vi "Cell colour.vi"() -> ()   [LabVIEW 2011]
uses:
  <vilib>/Utility/miscctls.llb/LVRowAndColumnTypeDef.ctl
panel:
  in  "Sub-Cycle Pattern":string[][](table) caption="Subcycle pattern"
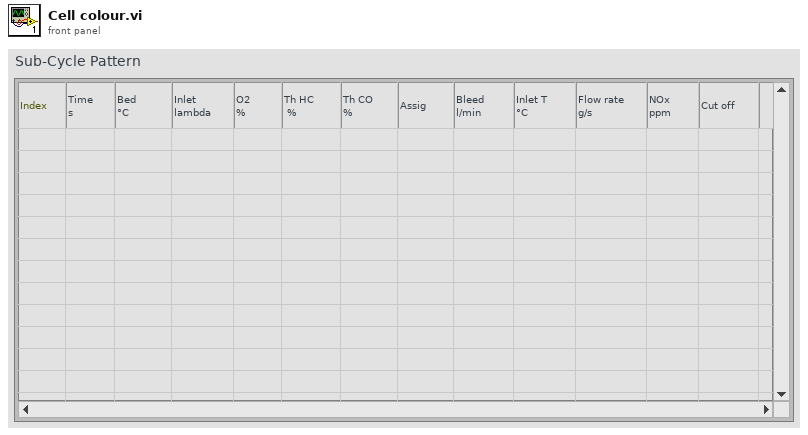
[diagram p1: front panel]
types:
  T1 = typedef "LVRowAndColumnTypeDef.ctl" = cluster{"Row":i32, "Column":i32}
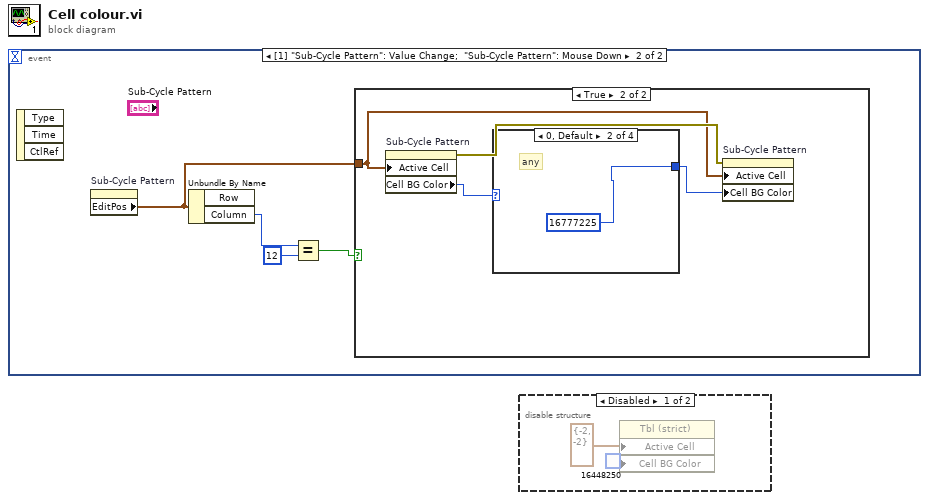
[diagram p0: block diagram]
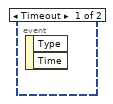
[diagram p3: hidden frame]
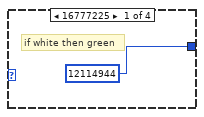
[diagram p5: hidden frame]
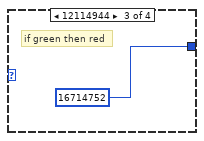
[diagram p6: hidden frame]
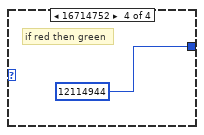
[diagram p7: hidden frame]
diagram:
  n1 = event shown="[1] \"Sub-Cycle Pattern\": Value Change;  \"Sub-Cycle Pattern\": Mouse Down" {
    selector: _ -> [_ _]
    dyn-events: _ -> [_ _]
    timeout: _ -> [_ _]
    event Timeout {
      n2 = event-data() -> ()  [unwired: 1 in, 2 out]
    }
    event "Sub-Cycle Pattern": Value Change; "Sub-Cycle Pattern": Mouse Down {
      n3 = event-data() -> ()  [unwired: 1 in, 3 out]
      n4 = property on="Sub-Cycle Pattern" class="Tbl (strict)"() -> ("EditPos"=w1:T1)  [unwired: 2 in, 2 out]
      n5 = Unbundle By Name(w1) -> ("Column"=w4:i32)  [unwired: 1 out]
      n6 = Equal?(x=w4, y=12) -> (x = y?=w2:bool)
      n7 = case shown="True" w2 {
        tunnel: w1 -> [_ w5]
        frame False {
        }
        frame True {
          n8 = property on="Sub-Cycle Pattern" class="Tbl (strict)"("Active Cell"=w5) -> (error out=w6:errorcluster, "Cell BG Color"=w7:u32)  [unwired: 2 in, 1 out]
          n9 = case shown="0, Default" w7 {
            tunnel: [12114944 ("y") 16777225 ("y") 16714752 ("y") 12114944 ("y")] -> w8
            frame 16777225 {
              # "if white then green"
            }
            frame 0, Default {
              # "any"
            }
            frame 12114944 {
              # "if green then red"
            }
            frame 16714752 {
              # "if red then green"
            }
          }
          n10 = property on="Sub-Cycle Pattern" class="Tbl (strict)"(error in=w6, "Active Cell"=w5, "Cell BG Color"=w8) -> ()  [unwired: 1 in, 2 out]
        }
      }
    }
  }
  n11 = disable-structure shown="Disabled" {
    frame Disabled {
      n12 = property on="Property Node" class="Tbl (strict)"("Active Cell"=T1 {"Row"=-2, "Column"=-2} ("Active Cell:Active Cell"), "Cell BG Color"=u32 16448250) -> ()  [unwired: 2 in, 2 out]
    }
    frame Enabled {
    }
  }
